vi "Write Instrument address.vi"(8 "error in (no error)":errorcluster, 10 "VISA address":refnum<visa-resource-name>, 11 "InstControl in":refnum<class "InstrControl.lvclass">) -> (0 "error out":errorcluster, 3 "InstControl out":refnum<class "InstrControl.lvclass">)   [LabVIEW 2013, in "InstrControl.lvclass"]
uses:
  InstrControl.lvclass
  InstrControl.lvclass/InstrControl.ctl
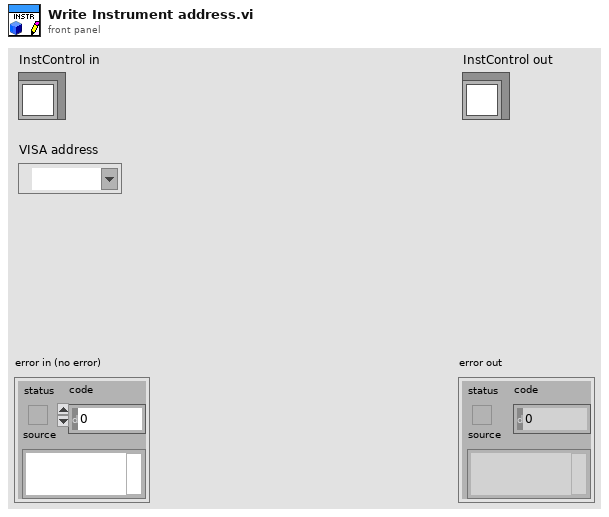
[diagram p1: front panel]
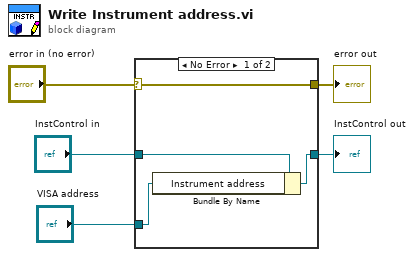
[diagram p0: block diagram]
diagram:
  n1 = case shown="No Error" "error in (no error)" {
    selector: "error in (no error)" -> [w9 w10]
    tunnel: [w9 w10] -> w4
    tunnel: [w7 w11] -> w2
    tunnel: "InstControl in" -> [w8 w11]
    tunnel: "VISA address" -> [w6 _]
    frame No Error {
      n2 = Bundle By Name(cluster=w8, "Instrument address"=w6) -> (w7:refnum<class "InstrControl.lvclass">)
    }
    frame Error {
    }
  }
  "error out" <- w4
  "InstControl out" <- w2
